vi "DAQ_Cnt_Open.vi"(0 "reference in":refnum<class "NI_DAQ.lvclass">, 5 "error in (no error)":errorcluster) -> (14 "reference out":refnum<class "NI_DAQ.lvclass">, 19 "error out":errorcluster)   [LabVIEW 2020, in "NI_DAQ.lvclass"]
uses:
  NI_DAQ.lvclass
panel:
  out "counter_task_out":refnum<k21>[](array[refnum])
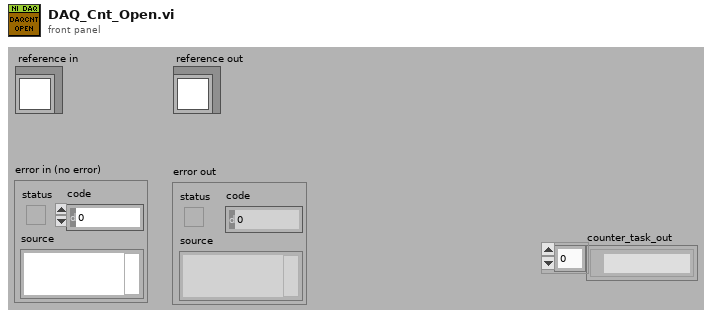
[diagram p1: front panel]
types:
  T1 = typedef "DAQ_Base.lvclass/DAQSettings.ctl" = cluster{"SampleSettings":T2, "AI_ChannelSettings":T3, "AO_ChannelSettings":T5, "Cnt_ChannelSettings":T6}
  T2 = typedef "DAQ_Base.lvclass/SampleSettings.ctl" = cluster{"samples per channel":i32, "SampleRate":dbl, "TansMaxLength":dbl, "ReadTimeOut":dbl, "时钟源":tag}
  T3 = typedef "DAQ_Base.lvclass/AI_ChannelSettings.ctl" = cluster{"AI_SettingsArry":cluster{"DeviceName":tag, "physical channels":tag, "AssignName":string, "输入信号类型":T4, "Max_value":dbl, "Min_value":dbl, "单位":i32, "shunt resistor location":i32, "external shunt resistor value":dbl, "标定系数":cluster{"Scale":dbl, "Offset":dbl}}[]}
  T4 = typedef "AI信号类型.ctl" = i32
  T5 = typedef "DAQ_Base.lvclass/AO_ChannelSettings.ctl" = cluster{"布尔":bool}
  T6 = typedef "DAQ_Base.lvclass/Cnt_ChannelSettings.ctl" = cluster{"Cnt_ChannelSettings":cluster{"类型":enum16{"Linear", "Rotate"}, "CounterNbr":tag, "AssignName":string, "单位":u16, "decoding type":u16, "PPR_DistancePerPulse":dbl, "Initial Position ":dbl, "z index enable":bool, "z index phase":i32, "source":tag}[]}
  T7 = typedef "NI_DAQ.lvclass/ObjectAttributesRef.ctl" = refnum<data-value>
  T8 = typedef "NI_DAQ.lvclass/ObjectAttributes.ctl" = cluster{"MyAttribute":dbl, "DAQ_AI_task_out":refnum<k21>, "counter_task_out":refnum<k21>[]}
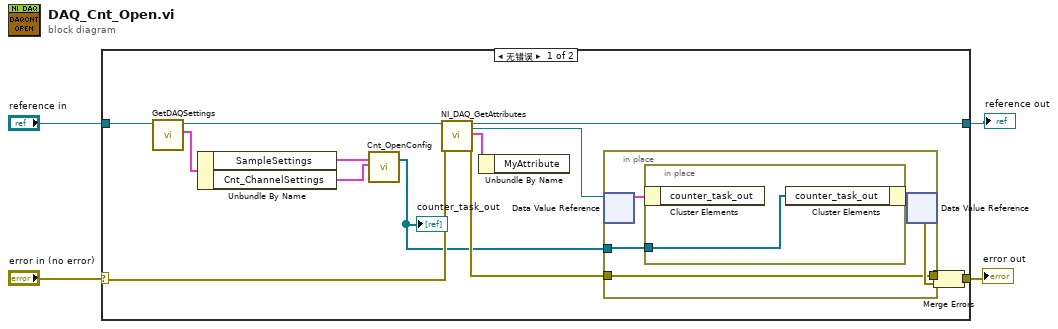
[diagram p0: block diagram]
diagram:
  n1 = case shown="无错误" "error in (no error)" {
    selector: "error in (no error)" -> [w15 w25]
    tunnel: [w18 w25] -> w3
    tunnel: [w16 w24] -> w1
    tunnel: "reference in" -> [w17 w24]
    frame No Error {
      n2 = call-dynamic "GetDAQSettings.vi"("reference in"=w17) -> ("DAQSettings"=w8:T1, "reference out"=w9:refnum<class "NI_DAQ.lvclass">)  [unwired: 8 in, 1 out]
      n3 = Unbundle By Name(w8) -> ("SampleSettings"=w7:T2, "Cnt_ChannelSettings"=w6:T6)
      n4 = call "Cnt_OpenConfig.vi"("SampleSettings"=w7, "Cnt_ChannelSettings"=w6) -> ("counter_task_out"=w5:refnum<k21>[])  [unwired: 16 in, 1 out]
      "counter_task_out" <- w5
      n5 = call "NI_DAQ_GetAttributes.vi"("reference in"=w9, "error in (no error)"=w15) -> ("reference out"=w16:refnum<class "NI_DAQ.lvclass">, "attributes ref"=w10:T7, "attributes"=w13:T8, "error out"=w14:errorcluster)  [unwired: 14 in]
      n6 = Unbundle By Name(w13) -> ()  [unwired: 1 out]
      n7 = in-place {
        in-place-border: w14 -> [w20]
        in-place-border: [w20] -> w12
        in-place-border: w5 -> [w19]
        n8 = in-place-dvr #1(w10) -> (w21:T8)  [unwired: 1 out]
        n9 = in-place {
          in-place-border: w19 -> [w23]
          n10 = in-place-cluster #2(w21) -> ()  [unwired: 1 out]
          n11 = in-place-cluster #2("counter_task_out"=w23) -> (w22:T8)
        }
        n12 = in-place-dvr #1(w22) -> (w11:errorcluster)  [unwired: 1 out]
      }
      n13 = Merge Errors(w12, w11) -> (w18:errorcluster)
    }
    frame Error {
    }
  }
  "error out" <- w3
  "reference out" <- w1
